vi "labview_port_of_shader.vi"(6 "Aberration":dbl[][](graph), 7 "Settings":T1, 9 "Total Intensity":dbl, 10 "Hologram Resolution":i32=1080, 11 "Spots":T2(array[cluster])=[{"X tilt"=0.0, "Y tilt"=0.0, "Z shift"=0.0, "L (vortex)"=0.0, "Phase Shift"=0.0, "Intensity"=1.0}]) -> (3 "Hologram (blazed, 0...1)":dbl[][](graph))   [LabVIEW 2010]
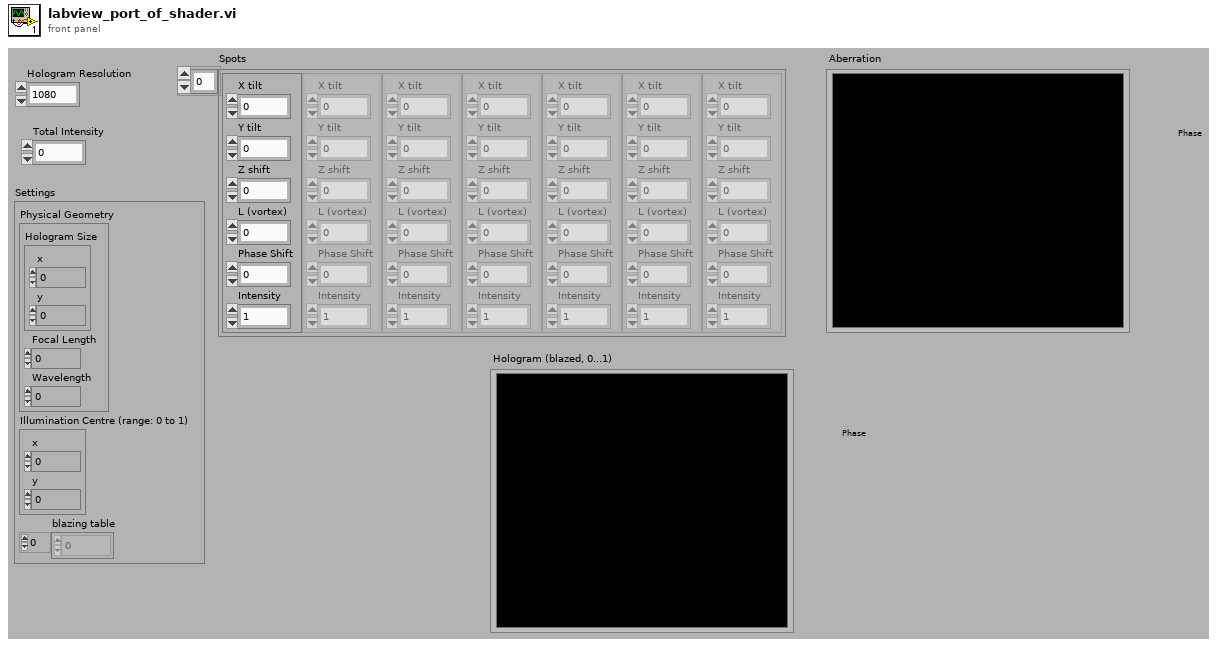
[diagram p1: front panel]
types:
  T1 = cluster{"Physical Geometry":cluster{"Hologram Size":cluster{"x":dbl, "y":dbl}, "Focal Length":dbl, "Wavelength":dbl}, "Illumination Centre (range: 0 to 1)":cluster{"x":dbl, "y":dbl}, "blazing table":dbl[]}
  T2 = cluster{"X tilt":dbl, "Y tilt":dbl, "Z shift":dbl, "L (vortex)":dbl, "Phase Shift":dbl, "Intensity":dbl}[]
  T3 = cluster{"Hologram Size":cluster{"x":dbl, "y":dbl}, "Focal Length":dbl, "Wavelength":dbl}
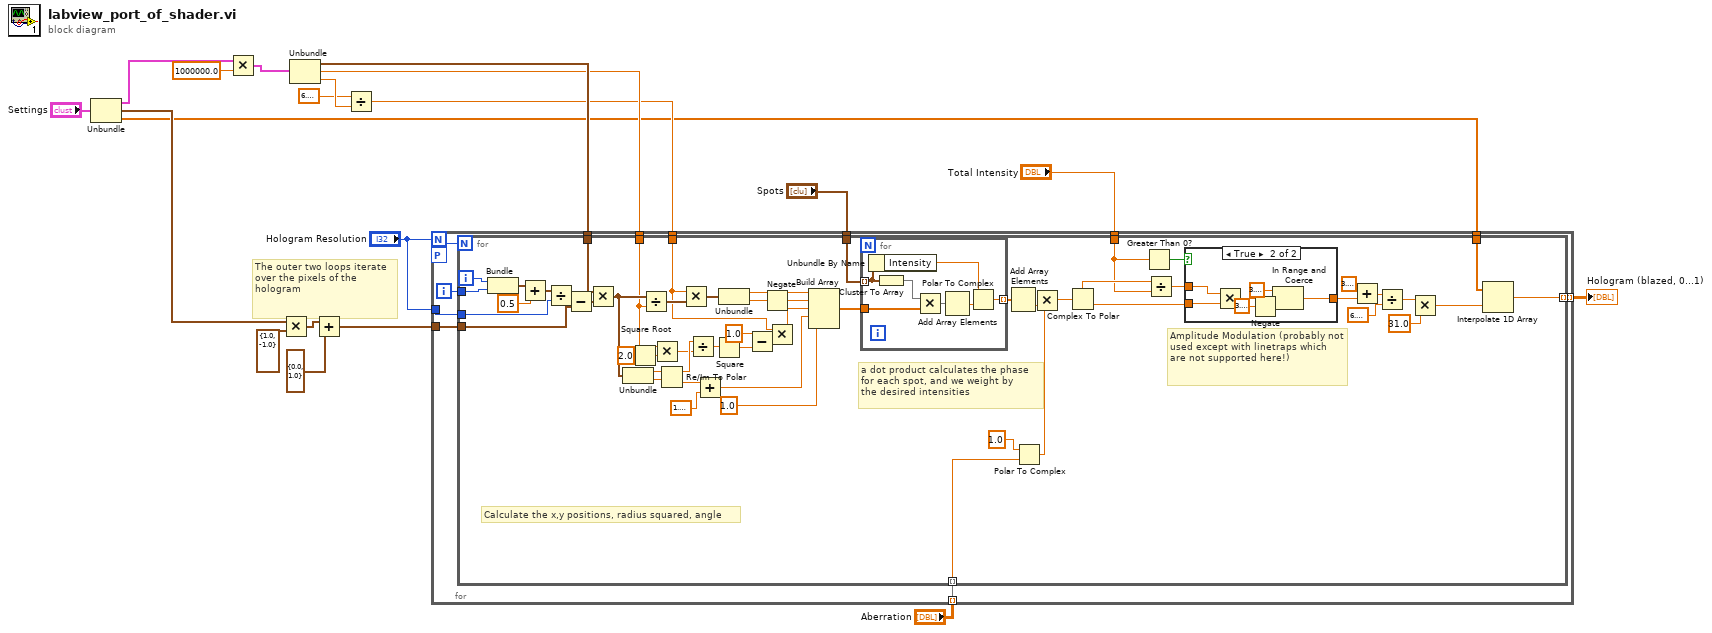
[diagram p0: block diagram]
diagram:
  # "The outer two loops iterate over the pixels of the hologram"
  n1 = Unbundle("Settings") -> ("Physical Geometry"=w13:T3, "Illumination Centre (range: 0 to 1)"=w9:cluster{"x":dbl, "y":dbl}, "blazing table"=w7:dbl[])
  n2 = Multiply(x=w13, y=1000000.0 ("Wavevector (2pi/wavelength)")) -> (x*y=w16:T3)
  n3 = Multiply(x=w9, y=cluster{"x":dbl, "y":dbl} {"x"=1.0, "y"=-1.0}) -> (x*y=w4:cluster{"x":dbl, "y":dbl})
  n4 = Unbundle(w16) -> ("Hologram Size"=w12:cluster{"x":dbl, "y":dbl}, "Focal Length"=w11:dbl, "Wavelength"=w15:dbl)
  n5 = Add(x=w4, y=cluster{"x":dbl, "y":dbl} {"x"=0.0, "y"=1.0} ("x")) -> (x+y=w2:cluster{"x":dbl, "y":dbl})
  n6 = Divide(x=6.283185307179586, y=w15) -> (x/y=w10:dbl)
  n7 = for {
    N: "Hologram Resolution" -> [w32]
    tunnel: "Hologram Resolution" -> [w30]
    tunnel: "Spots" -> [w29]
    workers-P: _ -> [_]
    tunnel: w12 -> [w28]
    tunnel: w11 -> [w27]
    tunnel: w10 -> [w26]
    tunnel: w2 -> [w25]
    tunnel: "Total Intensity" -> [w24]
    tunnel: w7 -> [w23]
    tunnel: [w22] -> w6 mode=indexing
    tunnel: "Aberration" -> [w21] mode=indexing
    i -> [w31]
    n8 = for {
      N: w32 -> [_]
      tunnel: w31 -> [w39]
      tunnel: w30 -> [w86]
      tunnel: w29 -> [w82]
      tunnel: w28 -> [w70]
      tunnel: w27 -> [w36]
      tunnel: w26 -> [w35]
      tunnel: w25 -> [w67]
      tunnel: w24 -> [w62]
      tunnel: w23 -> [w54]
      tunnel: [w53] -> w22 mode=indexing
      tunnel: w21 -> [w44] mode=indexing
      i -> [w40]
      # "Amplitude Modulation (probably not used except with linetraps which are not supported here!)"
      # "a dot product calculates the phase\nfor each spot, and we weight by\nthe desired intensities"
      # "Calculate the x,y positions, radius squared, angle"
      n9 = Bundle(w40, w39) -> (w87:cluster{i32, i32})  [unwired: 1 in]
      n10 = Add(x=w87, y=0.5) -> (x+y=w73:cluster{dbl, dbl})
      n11 = Divide(x=w73, y=w86) -> (x/y=w80:cluster{dbl, dbl})
      n12 = Subtract(x=w80, y=w67) -> (x-y=w74:cluster{dbl, dbl})
      n13 = Multiply(x=w70, y=w74) -> (x*y=w71:cluster{dbl, dbl})
      n14 = Unbundle(w71) -> (w78:dbl, w77:dbl)
      n15 = Square Root(x=2.0 ("y")) -> (sqrt(x)=w48:dbl)
      n16 = Divide(x=w71, y=w36) -> (x/y=w69:cluster{dbl, dbl})
      n17 = Multiply(x=w36, y=w48) -> (x*y=w50:dbl)
      n18 = Re/Im To Polar(2:w77, 3:w78) -> (0:w76:dbl, 1:w51:dbl)
      n19 = Multiply(x=w35, y=w69) -> (x*y=w68:cluster{dbl, dbl})
      n20 = Divide(x=w51, y=w50) -> (x/y=w47:dbl)
      n21 = Add(x=w76, y=1.5707963267948966) -> (x+y=w34:dbl)
      n22 = Square(x=w47) -> (x^2=w43:dbl)
      n23 = Unbundle(w68) -> (w85:dbl, w84:dbl)
      n24 = Subtract(x=sgl 1.0 ("element"), y=w43) -> (x-y=w41:dbl)
      n25 = Negate(x=w84) -> (-x=w38:dbl)
      n26 = Multiply(x=w35, y=w41) -> (x*y=w37:dbl)
      n27 = Build Array(w85, w38, w37, w34, sgl 1.0 ("element")) -> (w83:dbl[])
      n28 = for {
        tunnel: w83 -> [w102]
        tunnel: w82 -> [w97] mode=indexing
        tunnel: [w99] -> w81 mode=indexing
        n29 = Unbundle By Name(w97) -> ("Intensity"=w98:dbl)
        n30 = Cluster To Array(cluster=w97) -> (array=w96:dbl[])
        n31 = Multiply(x=w96, y=w102) -> (x*y=w101:dbl[])
        n32 = Add Array Elements(numeric array=w101) -> (sum=w100:dbl)
        n33 = Polar To Complex(1:w100, 2:w98) -> (0:w99:cdb)
      }
      n34 = Add Array Elements(numeric array=w81) -> (sum=w79:cdb)
      n35 = Polar To Complex(1:w44, 2:sgl 1.0 ("element")) -> (0:w45:cdb)
      n36 = Multiply(x=w45, y=w79) -> (x*y=w46:cdb)
      n37 = Complex To Polar(r * e^(i*theta)=w46) -> (r=w63:dbl, theta=w64:dbl)
      n38 = Greater Than 0?(x=w62) -> (x > 0?=w66:bool)
      n39 = Divide(x=w63, y=w62) -> (x/y=w65:dbl)
      n40 = case shown="True" w66 {
        tunnel: w64 -> [w88 w95]
        tunnel: w65 -> [_ w94]
        tunnel: [w88 w92] -> w61
        frame False {
        }
        frame True {
          n41 = Multiply(x=w94, y=w95) -> (x*y=w93:dbl)
          n42 = Negate(x=3.141592653589793) -> (-x=w89:dbl)
          n43 = In Range and Coerce(upper limit=3.141592653589793, x=w93, lower limit=w89) -> (coerced(x)=w92:dbl)  [unwired: 1 out]
        }
      }
      n44 = Add(x=3.141592653589793, y=w61) -> (x+y=w60:dbl)
      n45 = Divide(x=w60, y=6.283185307179586) -> (x/y=w57:dbl)
      n46 = Multiply(x=w57, y=31.0) -> (x*y=w55:dbl)
      n47 = Interpolate 1D Array(1:w55, 2:w54) -> (0:w53:dbl)
    }
  }
  "Hologram (blazed, 0...1)" <- w6
